vi "CALC_TRAN_TIME_MARK_MODE.vi"(0 "VISA IN":refnum<visa-resource-name>, 1 "MODE":string(combo), 5 "error in":errorcluster, 7 "Channel":i32) -> (14 "VISA Out":refnum<visa-resource-name>, 19 "error out":errorcluster)   [LabVIEW 2018, in "PNA-X.lvlib"]
doc: "CALCulate<cnum>:TRANsform:TIME:MARKer:MODE <char> \n(Read-Write) Specifies the measurement type in order to determine the correct marker distance. \nSelect Auto for S-Parameter measurements. \nSelect Reflection or Transmission for arbitrary ratio or unratioed measurements. \nThis setting affects the display of ALL markers for only the ACTIVE measurement. \nLearn more about Distance Markers. \nSee Critical Note \nParameters \n<cnum> Channel number of the measurement. There must be a selected measurement \non that channel. If unspecified, <cnum> is set to 1. \n<char> Choose from: \nAUTO If the active measurement is an S-Parameter, automatically chooses \nreflection or transmission. If non S-Parameter measurements, reflection is \nchosen. \nREFLection Displays the distance from the source to the receiver divided by \ntwo (to compensate for the return trip.) \nTRANsmission Displays the distance from the source to the receiver. \nExamples CALC:TRAN:TIME:MARK:MODE REFL \ncalculate2:transform:time:marker:mode auto \nQuery Syntax CALCulate<cnum>:TRANsform:TIME:MARKer:MODE? \n1569\n\nReturn Type Character \nDefault Auto"
uses:
  PNA-X.lvlib
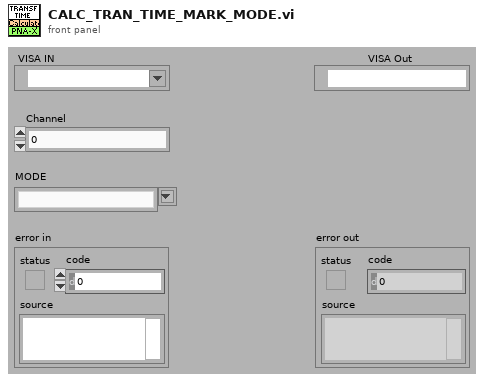
[diagram p1: front panel]
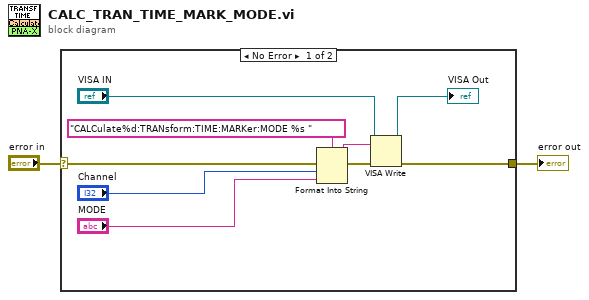
[diagram p0: block diagram]
diagram:
  n1 = case shown="No Error" "error in" {
    selector: "error in" -> [w11 w12]
    tunnel: [w6 w12] -> w1
    frame No Error {
      n2 = Format Into String(format string="CALCulate%d:TRANsform:TIME:MARKer:MODE %s " ("Cmdline"), error in=w11, "Channel", "MODE") -> (resulting string=w9:string, error out=w10:errorcluster)  [unwired: 1 in]
      n3 = VISA Write(VISA resource name="VISA IN", write buffer=w9, error in (no error)=w10) -> (VISA resource name out=→"VISA Out":refnum<visa-resource-name>, error out=w6:errorcluster)  [unwired: 1 out]
    }
    frame Error {
    }
  }
  "error out" <- w1
